vi "CLD 2  Elapsed Time Express Caller Exercise.vi"() -> ()   [LabVIEW 2009]
doc: "CLD 2 Exercise"
panel:
  out "Time Has Elapsed":bool
  out "Elapsed Time (s)":dbl format="%#.2g"
  out "error out":errorcluster
  in  "Time Target (s)":dbl
  in  "Auto Reset (F)":bool
  in  "error in (no error)":errorcluster
  in  "Timer Mode":enum16{"Reset", "Read Status", "Set Auto Reset"}(ring)
  in  "stop":bool
  # "Caller for the FGV"
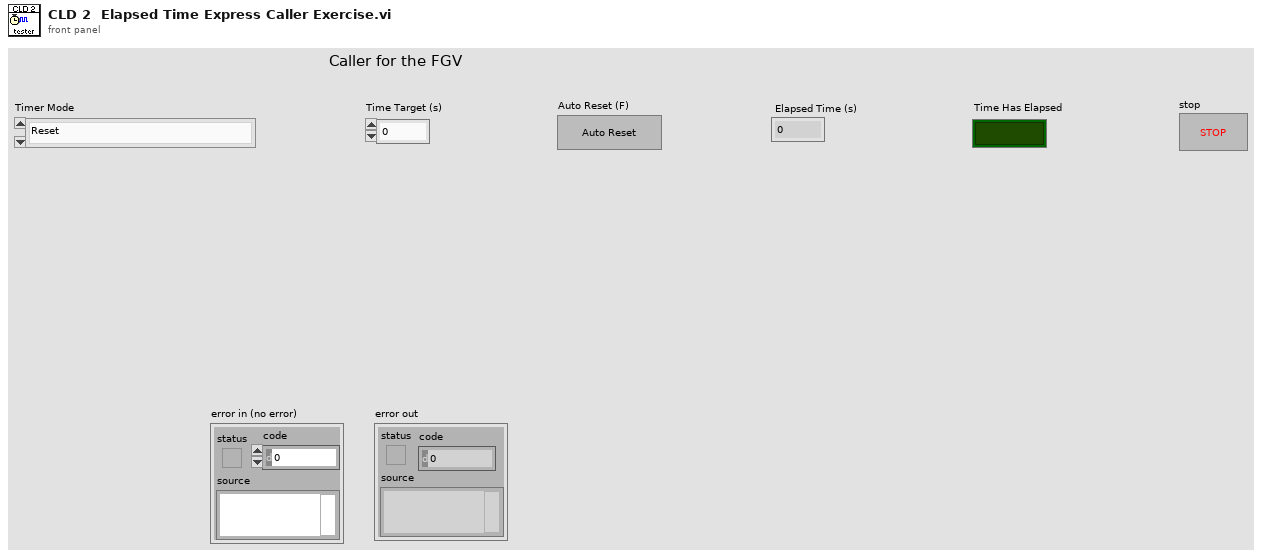
[diagram p1: front panel]
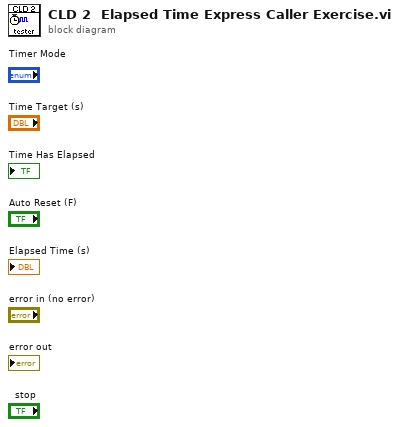
[diagram p0: block diagram]
diagram:
